vi "Read time.vi"(8 "error in (no error)":errorcluster, 11 "Test Results in":refnum<class "Test Results.lvclass">) -> (0 "error out":errorcluster, 2 "time / date":timestamp, 3 "Test Results out":refnum<class "Test Results.lvclass">)   [LabVIEW 2020, in "Test Results.lvclass"]
uses:
  Test Results.lvclass
  Test Results.lvclass/Test Results.ctl
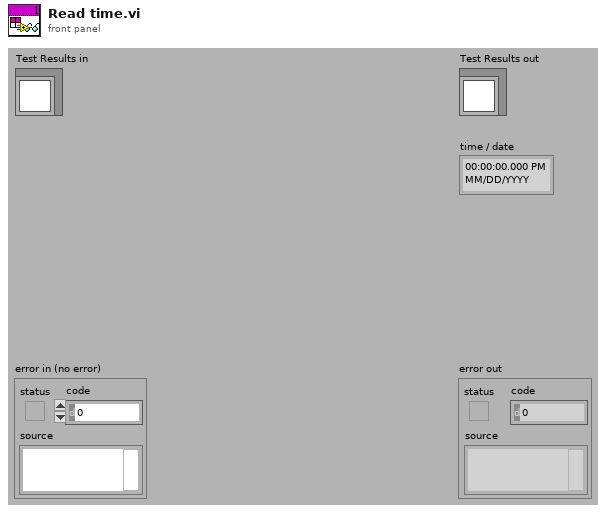
[diagram p1: front panel]
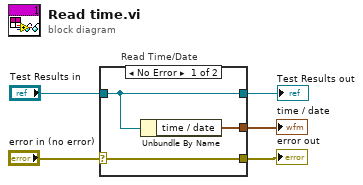
[diagram p0: block diagram]
diagram:
  # "Read Time/Date"
  n1 = case shown="No Error" "error in (no error)" {
    selector: "error in (no error)" -> [w8 w9]
    tunnel: [w8 w9] -> w4
    tunnel: [w7 w10] -> w2
    tunnel: "Test Results in" -> [w7 w10]
    tunnel: [w6 _] -> w1
    frame No Error {
      n2 = Unbundle By Name(w7) -> ("time / date"=w6:timestamp)
    }
    frame Error {
    }
  }
  "error out" <- w4
  "Test Results out" <- w2
  "time / date" <- w1
